vi "SP Convert 3.0 - 3.1 to 3.2 and 4.0 - 4.1.vi"(1 "S Parameter 3.0 - 3.1 Test Parameters":T2={"Tag"="", "Stimulus"={"Use Instrument Settings"=FALSE, "Sweep Type"=enum."Linear", "Sweep"=[{"Fstart, MHz"=500.0, "Fstop, MHz"=1500.0, "Points"=201}], "Blank Frequencies"=FALSE, "Power, dBm"=999.0, "IFBW, Hz"=-1.0, "Sweep Time, s"=-1.0}, "Measurements"=[{"Parameter"=enum."S11", "Channel"=1, "Limits"=[]}], "Reports"={"Reports to Generate"=[], "Print Reports"=FALSE}, "Quick Mode"=FALSE, "Display"={"Retain Settings"=FALSE, "Lock Control"=FALSE, "Plot Orientation"=enum."Single", "CH Controls"=[{"Trace Orientation"=enum."Overlay", "Frequency"={"Start"=500.0, "Stop"=1500.0, "Units"="MHz"}, "CH1Control"={"ChOn"=TRUE, "Measure"=0, "Format"=0, "Autoscale"=TRUE, "Reference"=0.0, "\nRefUnit"="dB/Div", "Position"=5.0, "Scale"=10.0, "ScaleUnit"="dB/Div", "LimitOn"=TRUE, "LimitFill"=FALSE, "Display Data"=0, "Show Markers"=FALSE}, "CH2Control"={"ChOn"=TRUE, "Measure"=0, "Format"=0, "Autoscale"=TRUE, "Reference"=0.0, "\nRefUnit"="dB/Div", "Position"=5.0, "Scale"=10.0, "ScaleUnit"="dB/Div", "LimitOn"=TRUE, "LimitFill"=FALSE, "Display Data"=0, "Show Markers"=FALSE}, "Markers"=[]}, {"Trace Orientation"=enum."Overlay", "Frequency"={"Start"=500.0, "Stop"=1500.0, "Units"="MHz"}, "CH1Control"={"ChOn"=TRUE, "Measure"=0, "Format"=0, "Autoscale"=TRUE, "Reference"=0.0, "\nRefUnit"="dB/Div", "Position"=5.0, "Scale"=10.0, "ScaleUnit"="dB/Div", "LimitOn"=TRUE, "LimitFill"=FALSE, "Display Data"=0, "Show Markers"=FALSE}, "CH2Control"={"ChOn"=TRUE, "Measure"=0, "Format"=0, "Autoscale"=TRUE, "Reference"=0.0, "\nRefUnit"="dB/Div", "Position"=5.0, "Scale"=10.0, "ScaleUnit"="dB/Div", "LimitOn"=TRUE, "LimitFill"=FALSE, "Display Data"=0, "Show Markers"=FALSE}, "Markers"=[]}, {"Trace Orientation"=enum."Overlay", "Frequency"={"Start"=500.0, "Stop"=1500.0, "Units"="MHz"}, "CH1Control"={"ChOn"=TRUE, "Measure"=0, "Format"=0, "Autoscale"=TRUE, "Reference"=0.0, "\nRefUnit"="dB/Div", "Position"=5.0, "Scale"=10.0, "ScaleUnit"="dB/Div", "LimitOn"=TRUE, "LimitFill"=FALSE, "Display Data"=0, "Show Markers"=FALSE}, "CH2Control"={"ChOn"=TRUE, "Measure"=0, "Format"=0, "Autoscale"=TRUE, "Reference"=0.0, "\nRefUnit"="dB/Div", "Position"=5.0, "Scale"=10.0, "ScaleUnit"="dB/Div", "LimitOn"=TRUE, "LimitFill"=FALSE, "Display Data"=0, "Show Markers"=FALSE}, "Markers"=[]}, {"Trace Orientation"=enum."Overlay", "Frequency"={"Start"=500.0, "Stop"=1500.0, "Units"="MHz"}, "CH1Control"={"ChOn"=TRUE, "Measure"=0, "Format"=0, "Autoscale"=TRUE, "Reference"=0.0, "\nRefUnit"="dB/Div", "Position"=5.0, "Scale"=10.0, "ScaleUnit"="dB/Div", "LimitOn"=TRUE, "LimitFill"=FALSE, "Display Data"=0, "Show Markers"=FALSE}, "CH2Control"={"ChOn"=TRUE, "Measure"=0, "Format"=0, "Autoscale"=TRUE, "Reference"=0.0, "\nRefUnit"="dB/Div", "Position"=5.0, "Scale"=10.0, "ScaleUnit"="dB/Div", "LimitOn"=TRUE, "LimitFill"=FALSE, "Display Data"=0, "Show Markers"=FALSE}, "Markers"=[]}], "Formatted Data"=FALSE}, "Calibrations"=[enum."Not Calibrated", enum."Not Calibrated", enum."Not Calibrated", enum."Not Calibrated"]} {"Stimulus"."Sweep Time, s" format="%.3g"; "Display"."CH Controls"."Frequency"."Stop" format="%.3g"; "Display"."CH Controls"."Frequency"."Start" format="%.3g"; "Display"."CH Controls"."CH2Control"."Measure" items=["S11", "S21", "S12", "S22"]; "Display"."CH Controls"."CH2Control"."Reference" format="%#.2g"; "Display"."CH Controls"."CH2Control"."Display Data" items=["Data", "Memory", "Data/Memory"]; "Display"."CH Controls"."CH2Control"."Format" items=["Log Mag", "Phase", "Delay", "Smith", "Polar", "Lin Mag", "SWR", "Loss", "Real", "Imaginary"]; "Display"."CH Controls"."CH2Control"."Scale" min=0.001 step=1.0 format="%#.2g"; "Display"."CH Controls"."CH2Control"."Position" min=0.0 max=10.0; "Display"."CH Controls"."CH1Control"."Measure" items=["S11", "S21", "S12", "S22"]; "Display"."CH Controls"."CH1Control"."Reference" format="%#.2g"; "Display"."CH Controls"."CH1Control"."Display Data" items=["Data", "Memory", "Data/Memory"]; "Display"."CH Controls"."CH1Control"."Format" items=["Log Mag", "Phase", "Delay", "Smith", "Polar", "Lin Mag", "SWR", "Loss", "Real", "Imaginary"]; "Display"."CH Controls"."CH1Control"."Scale" min=0.001 step=1.0 format="%#.2g"; "Display"."CH Controls"."CH1Control"."Position" min=0.0 max=10.0; "Measurements"."Channel" min=1 max=99 step=1; "Measurements"."Limits"."Run" min=1 step=1}) -> (0 "S Parameter 3.2 - 4.1 Test Parameters":T1={"Tag"="", "Stimulus"={"Use Instrument Settings"=FALSE, "Sweep Type"=enum."Linear", "Sweep"=[{"Fstart, MHz"=500.0, "Fstop, MHz"=1500.0, "Points"=201}], "Blank Frequencies"=FALSE, "Power, dBm"=999.0, "IFBW, Hz"=-1.0, "Sweep Time, s"=-1.0}, "Measurements"=[], "Datasheets"={"Datasheets to Generate"=[], "Print Datasheets"=FALSE}, "Quick Mode"=FALSE, "Display"={"Retain Settings"=TRUE, "Lock Control"=FALSE, "Plot Orientation"=enum."Single", "CH Controls"=[{"Trace Orientation"=enum."Overlay", "Frequency"={"Start"=500.0, "Stop"=1500.0, "Units"="MHz"}, "CH1Control"={"ChOn"=TRUE, "Measure"=0, "Format"=6, "Autoscale"=FALSE, "Reference"=0.0, "\nRefUnit"="dB/Div", "Position"=5.0, "Scale"=1.0, "ScaleUnit"="dB/Div", "LimitOn"=TRUE, "LimitFill"=FALSE, "Display Data"=0, "Show Markers"=FALSE, "SXX"=""}, "CH2Control"={"ChOn"=TRUE, "Measure"=0, "Format"=6, "Autoscale"=FALSE, "Reference"=0.0, "\nRefUnit"="dB/Div", "Position"=5.0, "Scale"=1.0, "ScaleUnit"="dB/Div", "LimitOn"=TRUE, "LimitFill"=FALSE, "Display Data"=0, "Show Markers"=FALSE, "SXX"=""}, "Markers"=[]}, {"Trace Orientation"=enum."Overlay", "Frequency"={"Start"=500.0, "Stop"=1500.0, "Units"="MHz"}, "CH1Control"={"ChOn"=TRUE, "Measure"=0, "Format"=6, "Autoscale"=TRUE, "Reference"=0.0, "\nRefUnit"="dB/Div", "Position"=5.0, "Scale"=1.0, "ScaleUnit"="dB/Div", "LimitOn"=TRUE, "LimitFill"=FALSE, "Display Data"=0, "Show Markers"=FALSE, "SXX"=""}, "CH2Control"={"ChOn"=TRUE, "Measure"=1, "Format"=0, "Autoscale"=TRUE, "Reference"=0.0, "\nRefUnit"="dB/Div", "Position"=5.0, "Scale"=1.0, "ScaleUnit"="dB/Div", "LimitOn"=TRUE, "LimitFill"=FALSE, "Display Data"=0, "Show Markers"=FALSE, "SXX"=""}, "Markers"=[]}, {"Trace Orientation"=enum."Overlay", "Frequency"={"Start"=500.0, "Stop"=1500.0, "Units"="MHz"}, "CH1Control"={"ChOn"=TRUE, "Measure"=0, "Format"=6, "Autoscale"=TRUE, "Reference"=0.0, "\nRefUnit"="dB/Div", "Position"=5.0, "Scale"=1.0, "ScaleUnit"="dB/Div", "LimitOn"=TRUE, "LimitFill"=FALSE, "Display Data"=0, "Show Markers"=FALSE, "SXX"=""}, "CH2Control"={"ChOn"=TRUE, "Measure"=1, "Format"=0, "Autoscale"=TRUE, "Reference"=0.0, "\nRefUnit"="dB/Div", "Position"=5.0, "Scale"=1.0, "ScaleUnit"="dB/Div", "LimitOn"=TRUE, "LimitFill"=FALSE, "Display Data"=0, "Show Markers"=FALSE, "SXX"=""}, "Markers"=[]}, {"Trace Orientation"=enum."Overlay", "Frequency"={"Start"=500.0, "Stop"=1500.0, "Units"="MHz"}, "CH1Control"={"ChOn"=TRUE, "Measure"=0, "Format"=6, "Autoscale"=TRUE, "Reference"=0.0, "\nRefUnit"="dB/Div", "Position"=5.0, "Scale"=1.0, "ScaleUnit"="dB/Div", "LimitOn"=TRUE, "LimitFill"=FALSE, "Display Data"=0, "Show Markers"=FALSE, "SXX"=""}, "CH2Control"={"ChOn"=TRUE, "Measure"=1, "Format"=0, "Autoscale"=TRUE, "Reference"=0.0, "\nRefUnit"="dB/Div", "Position"=5.0, "Scale"=1.0, "ScaleUnit"="dB/Div", "LimitOn"=TRUE, "LimitFill"=FALSE, "Display Data"=0, "Show Markers"=FALSE, "SXX"=""}, "Markers"=[]}], "Formatted Data"=FALSE}, "Auto Select"=TRUE, "Calibration"={"State"=FALSE, "String"=""}} {"Stimulus"."Sweep Time, s" format="%.3g"; "Display"."CH Controls"."Frequency"."Stop" format="%.3g"; "Display"."CH Controls"."Frequency"."Start" format="%.3g"; "Display"."CH Controls"."CH2Control"."Reference" format="%#.2g"; "Display"."CH Controls"."CH2Control"."Display Data" items=["Data", "Memory", "Data/Memory"]; "Display"."CH Controls"."CH2Control"."Format" items=["Log Mag", "Phase", "Delay", "Smith", "Polar", "Lin Mag", "SWR", "Loss", "Real", "Imaginary"]; "Display"."CH Controls"."CH2Control"."Scale" min=0.001 step=1.0 format="%#.2g"; "Display"."CH Controls"."CH2Control"."Position" min=0.0 max=10.0; "Display"."CH Controls"."CH1Control"."Reference" format="%#.2g"; "Display"."CH Controls"."CH1Control"."Display Data" items=["Data", "Memory", "Data/Memory"]; "Display"."CH Controls"."CH1Control"."Format" items=["Log Mag", "Phase", "Delay", "Smith", "Polar", "Lin Mag", "SWR", "Loss", "Real", "Imaginary"]; "Display"."CH Controls"."CH1Control"."Scale" min=0.001 step=1.0 format="%#.2g"; "Display"."CH Controls"."CH1Control"."Position" min=0.0 max=10.0; "Measurements"."Parameters"."Limits"."Run" min=1 step=1; "Measurements"."Channel" min=0 max=32 step=1})   [LabVIEW 2011]
uses:
  TypeDefs/SP Test Parameters v3.0-3.1.ctl
  TypeDefs/SP Test Parameters v3.2 and 4.0-4.1.ctl
  TypeDefs/SP Parameter.ctl
panel:
  # "Div"
  # "Div"
  # "="
  # "Div"
  # "Div"
  # "="
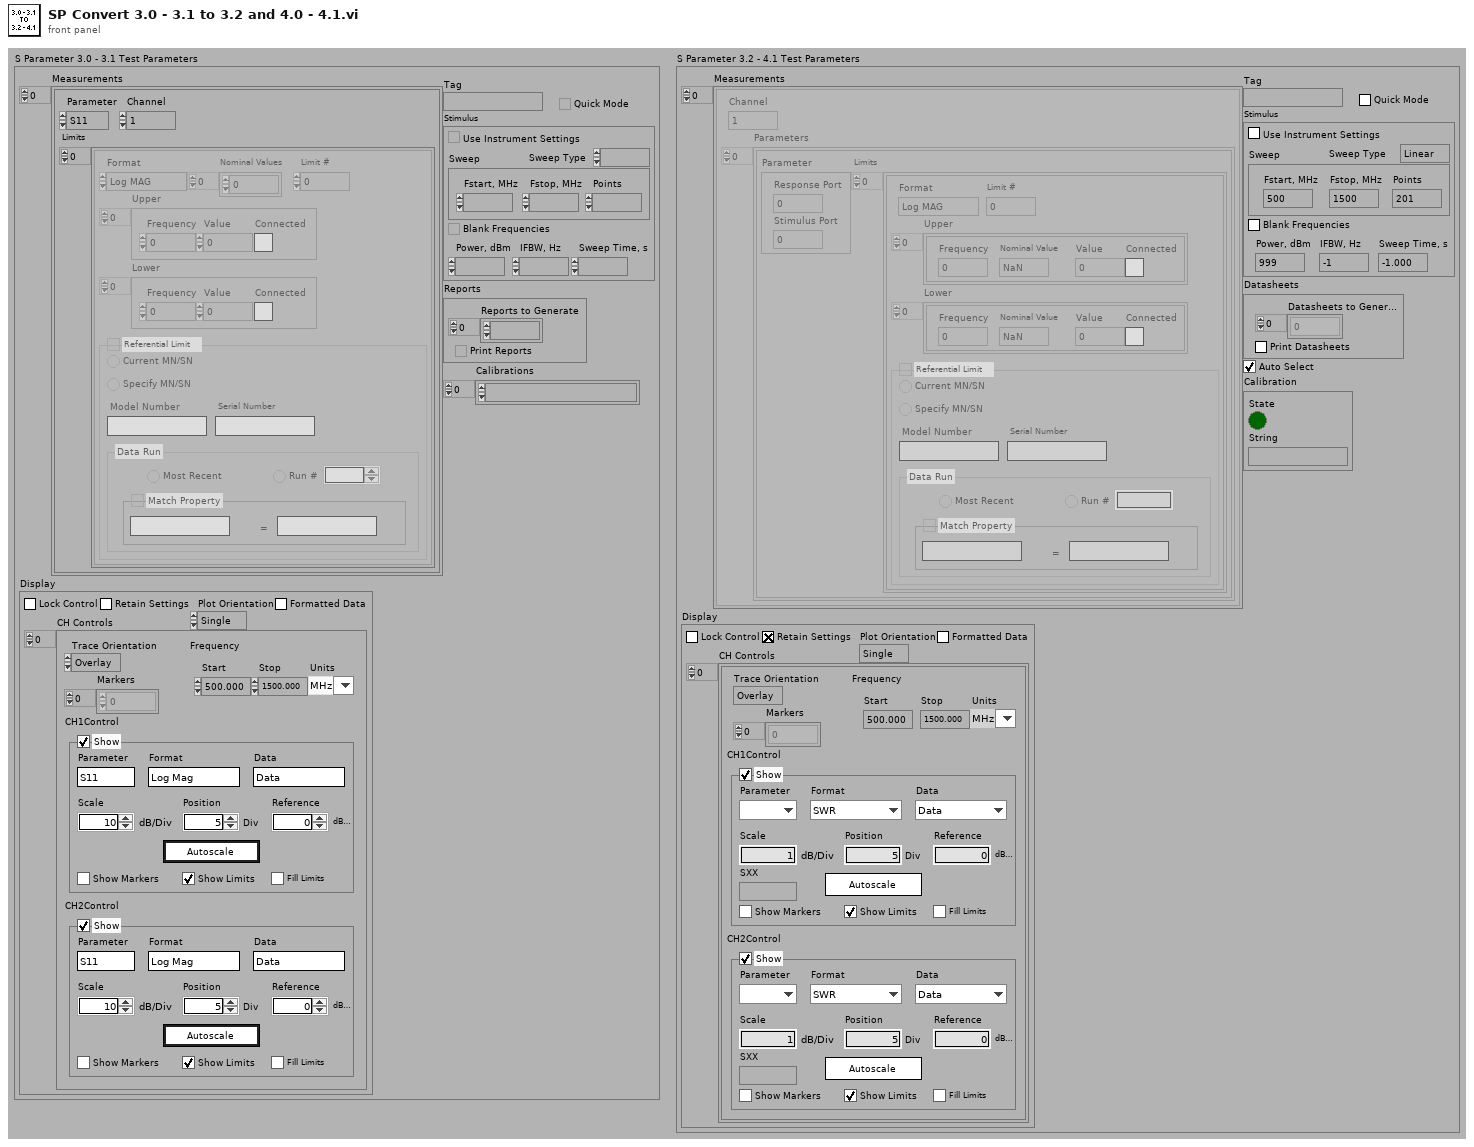
[diagram p1: front panel]
types:
  T1 = typedef "SP Test Parameters v3.2 and 4.0-4.1.ctl" = cluster{"Tag":string, "Stimulus":cluster{"Use Instrument Settings":bool, "Sweep Type":enum32{"Linear", "Log", "List", "Power", "CW"}, "Sweep":cluster{"Fstart, MHz":dbl, "Fstop, MHz":dbl, "Points":i32}[], "Blank Frequencies":bool, "Power, dBm":dbl, "IFBW, Hz":dbl, "Sweep Time, s":dbl}, "Measurements":cluster{"Channel":i8, "Parameters":cluster{"Parameter":cluster{"Stimulus Port":i8, "Response Port":i8}, "Limits":cluster{"Format":enum16{"Log MAG", "Lin MAG", "VSWR", "Phase", "Delay", "Insertion Loss", "Isolation", "Return Loss"}, "Upper":cluster{"Frequency":dbl, "Nominal Value":dbl, "Value":dbl, "Connected":bool}[], "Lower":cluster{"Frequency":dbl, "Nominal Value":dbl, "Value":dbl, "Connected":bool}[], "Limit #":i32, "Ref Limit":bool, "Ref Type":enum32{"Current", "Specify"}, "Model":string, "Serial":string, "Run Type":enum32{"Most Recent", "Run #"}, "Run":i32, "Match Property":bool, "Property":string, "Property Value":string}[]}[]}[], "Datasheets":cluster{"Datasheets to Generate":i32[], "Print Datasheets":bool}, "Quick Mode":bool, "Display":cluster{"Retain Settings":bool, "Lock Control":bool, "Plot Orientation":enum32{"Single", "Dual", "Quad"}, "CH Controls":cluster{"Trace Orientation":enum32{"Overlay", "Split"}, "Frequency":cluster{"Start":dbl, "Stop":dbl, "Units":string}, "CH1Control":cluster{"ChOn":bool, "Measure":i32, "Format":i32, "Autoscale":bool, "Reference":dbl, "\nRefUnit":string, "Position":dbl, "Scale":dbl, "ScaleUnit":string, "LimitOn":bool, "LimitFill":bool, "Display Data":u16, "Show Markers":bool, "SXX":string}, "CH2Control":cluster{"ChOn":bool, "Measure":i32, "Format":i32, "Autoscale":bool, "Reference":dbl, "\nRefUnit":string, "Position":dbl, "Scale":dbl, "ScaleUnit":string, "LimitOn":bool, "LimitFill":bool, "Display Data":u16, "Show Markers":bool, "SXX":string}, "Markers":dbl[]}[], "Formatted Data":bool}, "Auto Select":bool, "Calibration":cluster{"State":bool, "String":string}}
  T2 = typedef "SP Test Parameters v3.0-3.1.ctl" = cluster{"Tag":string, "Stimulus":cluster{"Use Instrument Settings":bool, "Sweep Type":enum32{"Linear", "Log", "List", "Power", "CW"}, "Sweep":cluster{"Fstart, MHz":dbl, "Fstop, MHz":dbl, "Points":i32}[], "Blank Frequencies":bool, "Power, dBm":dbl, "IFBW, Hz":dbl, "Sweep Time, s":dbl}, "Measurements":cluster{"Parameter":enum32{"S11", "S21", "S12", "S22"}, "Channel":i32, "Limits":cluster{"Format":enum16{"Log MAG", "Lin MAG", "VSWR", "Phase", "Delay", "Insertion Loss", "Isolation", "Return Loss"}, "Upper":cluster{"Frequency":dbl, "Value":dbl, "Connected":bool}[], "Lower":cluster{"Frequency":dbl, "Value":dbl, "Connected":bool}[], "Nominal Values":dbl[], "Limit #":i32, "Ref Limit":bool, "Ref Type":enum32{"Current", "Specify"}, "Model":string, "Serial":string, "Run Type":enum32{"Most Recent", "Run #"}, "Run":i32, "Match Property":bool, "Property":string, "Property Value":string}[]}[], "Reports":cluster{"Reports to Generate":i32[], "Print Reports":bool}, "Quick Mode":bool, "Display":cluster{"Retain Settings":bool, "Lock Control":bool, "Plot Orientation":enum32{"Single", "Dual", "Quad"}, "CH Controls":cluster{"Trace Orientation":enum32{"Overlay", "Split"}, "Frequency":cluster{"Start":dbl, "Stop":dbl, "Units":string}, "CH1Control":cluster{"ChOn":bool, "Measure":i32, "Format":i32, "Autoscale":bool, "Reference":dbl, "\nRefUnit":string, "Position":dbl, "Scale":dbl, "ScaleUnit":string, "LimitOn":bool, "LimitFill":bool, "Display Data":u16, "Show Markers":bool}, "CH2Control":cluster{"ChOn":bool, "Measure":i32, "Format":i32, "Autoscale":bool, "Reference":dbl, "\nRefUnit":string, "Position":dbl, "Scale":dbl, "ScaleUnit":string, "LimitOn":bool, "LimitFill":bool, "Display Data":u16, "Show Markers":bool}, "Markers":dbl[]}[], "Formatted Data":bool}, "Calibrations":enum32{"Not Calibrated", "Response", "Response and Isolation", "Full 1-Port (Port 1)", "Full 1-Port (Port 2)", "Full 2-Port", "One Path 2-Port", "TRL/LRM  2-Port", "TOSM Multi-Port", "TOM 2-Port", "TRM 2-Port", "TNA 2-Port"}[]}
  T3 = enum32{"Not Calibrated", "Response", "Response and Isolation", "Full 1-Port (Port 1)", "Full 1-Port (Port 2)", "Full 2-Port", "One Path 2-Port", "TRL/LRM  2-Port", "TOSM Multi-Port", "TOM 2-Port", "TRM 2-Port", "TNA 2-Port"}
  T4 = cluster{"Trace Orientation":enum32{"Overlay", "Split"}, "Frequency":cluster{"Start":dbl, "Stop":dbl, "Units":string}, "CH1Control":cluster{"ChOn":bool, "Measure":i32, "Format":i32, "Autoscale":bool, "Reference":dbl, "\nRefUnit":string, "Position":dbl, "Scale":dbl, "ScaleUnit":string, "LimitOn":bool, "LimitFill":bool, "Display Data":u16, "Show Markers":bool, "SXX":string}, "CH2Control":cluster{"ChOn":bool, "Measure":i32, "Format":i32, "Autoscale":bool, "Reference":dbl, "\nRefUnit":string, "Position":dbl, "Scale":dbl, "ScaleUnit":string, "LimitOn":bool, "LimitFill":bool, "Display Data":u16, "Show Markers":bool, "SXX":string}, "Markers":dbl[]}[]
  T5 = cluster{"Channel":i8, "Parameters":cluster{"Parameter":cluster{"Stimulus Port":i8, "Response Port":i8}, "Limits":cluster{"Format":enum16{"Log MAG", "Lin MAG", "VSWR", "Phase", "Delay", "Insertion Loss", "Isolation", "Return Loss"}, "Upper":cluster{"Frequency":dbl, "Nominal Value":dbl, "Value":dbl, "Connected":bool}[], "Lower":cluster{"Frequency":dbl, "Nominal Value":dbl, "Value":dbl, "Connected":bool}[], "Limit #":i32, "Ref Limit":bool, "Ref Type":enum32{"Current", "Specify"}, "Model":string, "Serial":string, "Run Type":enum32{"Most Recent", "Run #"}, "Run":i32, "Match Property":bool, "Property":string, "Property Value":string}[]}[]}[]
  T6 = cluster{"Use Instrument Settings":bool, "Sweep Type":enum32{"Linear", "Log", "List", "Power", "CW"}, "Sweep":cluster{"Fstart, MHz":dbl, "Fstop, MHz":dbl, "Points":i32}[], "Blank Frequencies":bool, "Power, dBm":dbl, "IFBW, Hz":dbl, "Sweep Time, s":dbl}
  T7 = cluster{"Reports to Generate":i32[], "Print Reports":bool}
  T8 = enum32{"Not Calibrated", "Response", "Response and Isolation", "Full 1-Port (Port 1)", "Full 1-Port (Port 2)", "Full 2-Port", "One Path 2-Port", "TRL/LRM  2-Port", "TOSM Multi-Port", "TOM 2-Port", "TRM 2-Port", "TNA 2-Port"}[]
  T9 = cluster{"Trace Orientation":enum32{"Overlay", "Split"}, "Frequency":cluster{"Start":dbl, "Stop":dbl, "Units":string}, "CH1Control":cluster{"ChOn":bool, "Measure":i32, "Format":i32, "Autoscale":bool, "Reference":dbl, "\nRefUnit":string, "Position":dbl, "Scale":dbl, "ScaleUnit":string, "LimitOn":bool, "LimitFill":bool, "Display Data":u16, "Show Markers":bool}, "CH2Control":cluster{"ChOn":bool, "Measure":i32, "Format":i32, "Autoscale":bool, "Reference":dbl, "\nRefUnit":string, "Position":dbl, "Scale":dbl, "ScaleUnit":string, "LimitOn":bool, "LimitFill":bool, "Display Data":u16, "Show Markers":bool}, "Markers":dbl[]}[]
  T10 = cluster{"Parameter":enum32{"S11", "S21", "S12", "S22"}, "Channel":i32, "Limits":cluster{"Format":enum16{"Log MAG", "Lin MAG", "VSWR", "Phase", "Delay", "Insertion Loss", "Isolation", "Return Loss"}, "Upper":cluster{"Frequency":dbl, "Value":dbl, "Connected":bool}[], "Lower":cluster{"Frequency":dbl, "Value":dbl, "Connected":bool}[], "Nominal Values":dbl[], "Limit #":i32, "Ref Limit":bool, "Ref Type":enum32{"Current", "Specify"}, "Model":string, "Serial":string, "Run Type":enum32{"Most Recent", "Run #"}, "Run":i32, "Match Property":bool, "Property":string, "Property Value":string}[]}[]
  T11 = cluster{"Channel":i8, "Parameters":cluster{"Parameter":cluster{"Stimulus Port":i8, "Response Port":i8}, "Limits":cluster{"Format":enum16{"Log MAG", "Lin MAG", "VSWR", "Phase", "Delay", "Insertion Loss", "Isolation", "Return Loss"}, "Upper":cluster{"Frequency":dbl, "Nominal Value":dbl, "Value":dbl, "Connected":bool}[], "Lower":cluster{"Frequency":dbl, "Nominal Value":dbl, "Value":dbl, "Connected":bool}[], "Limit #":i32, "Ref Limit":bool, "Ref Type":enum32{"Current", "Specify"}, "Model":string, "Serial":string, "Run Type":enum32{"Most Recent", "Run #"}, "Run":i32, "Match Property":bool, "Property":string, "Property Value":string}[]}[]}
  T12 = cluster{"Parameter":cluster{"Stimulus Port":i8, "Response Port":i8}, "Limits":cluster{"Format":enum16{"Log MAG", "Lin MAG", "VSWR", "Phase", "Delay", "Insertion Loss", "Isolation", "Return Loss"}, "Upper":cluster{"Frequency":dbl, "Nominal Value":dbl, "Value":dbl, "Connected":bool}[], "Lower":cluster{"Frequency":dbl, "Nominal Value":dbl, "Value":dbl, "Connected":bool}[], "Limit #":i32, "Ref Limit":bool, "Ref Type":enum32{"Current", "Specify"}, "Model":string, "Serial":string, "Run Type":enum32{"Most Recent", "Run #"}, "Run":i32, "Match Property":bool, "Property":string, "Property Value":string}[]}[]
  T13 = cluster{"Trace Orientation":enum32{"Overlay", "Split"}, "Frequency":cluster{"Start":dbl, "Stop":dbl, "Units":string}, "CH1Control":cluster{"ChOn":bool, "Measure":i32, "Format":i32, "Autoscale":bool, "Reference":dbl, "\nRefUnit":string, "Position":dbl, "Scale":dbl, "ScaleUnit":string, "LimitOn":bool, "LimitFill":bool, "Display Data":u16, "Show Markers":bool, "SXX":string}, "CH2Control":cluster{"ChOn":bool, "Measure":i32, "Format":i32, "Autoscale":bool, "Reference":dbl, "\nRefUnit":string, "Position":dbl, "Scale":dbl, "ScaleUnit":string, "LimitOn":bool, "LimitFill":bool, "Display Data":u16, "Show Markers":bool, "SXX":string}, "Markers":dbl[]}
  T14 = typedef "SP Display Data.ctl" = u16
  T15 = cluster{"Parameter":cluster{"Stimulus Port":i8, "Response Port":i8}, "Limits":cluster{"Format":enum16{"Log MAG", "Lin MAG", "VSWR", "Phase", "Delay", "Insertion Loss", "Isolation", "Return Loss"}, "Upper":cluster{"Frequency":dbl, "Nominal Value":dbl, "Value":dbl, "Connected":bool}[], "Lower":cluster{"Frequency":dbl, "Nominal Value":dbl, "Value":dbl, "Connected":bool}[], "Limit #":i32, "Ref Limit":bool, "Ref Type":enum32{"Current", "Specify"}, "Model":string, "Serial":string, "Run Type":enum32{"Most Recent", "Run #"}, "Run":i32, "Match Property":bool, "Property":string, "Property Value":string}[]}
  T16 = cluster{"Format":enum16{"Log MAG", "Lin MAG", "VSWR", "Phase", "Delay", "Insertion Loss", "Isolation", "Return Loss"}, "Upper":cluster{"Frequency":dbl, "Nominal Value":dbl, "Value":dbl, "Connected":bool}[], "Lower":cluster{"Frequency":dbl, "Nominal Value":dbl, "Value":dbl, "Connected":bool}[], "Limit #":i32, "Ref Limit":bool, "Ref Type":enum32{"Current", "Specify"}, "Model":string, "Serial":string, "Run Type":enum32{"Most Recent", "Run #"}, "Run":i32, "Match Property":bool, "Property":string, "Property Value":string}[]
  T17 = cluster{"Format":enum16{"Log MAG", "Lin MAG", "VSWR", "Phase", "Delay", "Insertion Loss", "Isolation", "Return Loss"}, "Upper":cluster{"Frequency":dbl, "Nominal Value":dbl, "Value":dbl, "Connected":bool}[], "Lower":cluster{"Frequency":dbl, "Nominal Value":dbl, "Value":dbl, "Connected":bool}[], "Limit #":i32, "Ref Limit":bool, "Ref Type":enum32{"Current", "Specify"}, "Model":string, "Serial":string, "Run Type":enum32{"Most Recent", "Run #"}, "Run":i32, "Match Property":bool, "Property":string, "Property Value":string}
  T18 = cluster{"Frequency":dbl, "Nominal Value":dbl, "Value":dbl, "Connected":bool}[]
  T19 = cluster{"Frequency":dbl, "Nominal Value":dbl, "Value":dbl, "Connected":bool}
  T20 = typedef "SP Parameter.ctl" = cluster{"Stimulus Port":i8, "Response Port":i8}
  T21 = cluster{"Format":enum16{"Log MAG", "Lin MAG", "VSWR", "Phase", "Delay", "Insertion Loss", "Isolation", "Return Loss"}, "Upper":cluster{"Frequency":dbl, "Value":dbl, "Connected":bool}[], "Lower":cluster{"Frequency":dbl, "Value":dbl, "Connected":bool}[], "Nominal Values":dbl[], "Limit #":i32, "Ref Limit":bool, "Ref Type":enum32{"Current", "Specify"}, "Model":string, "Serial":string, "Run Type":enum32{"Most Recent", "Run #"}, "Run":i32, "Match Property":bool, "Property":string, "Property Value":string}[]
  T22 = enum16{"Log MAG", "Lin MAG", "VSWR", "Phase", "Delay", "Insertion Loss", "Isolation", "Return Loss"}
  T23 = cluster{"Frequency":dbl, "Value":dbl, "Connected":bool}[]
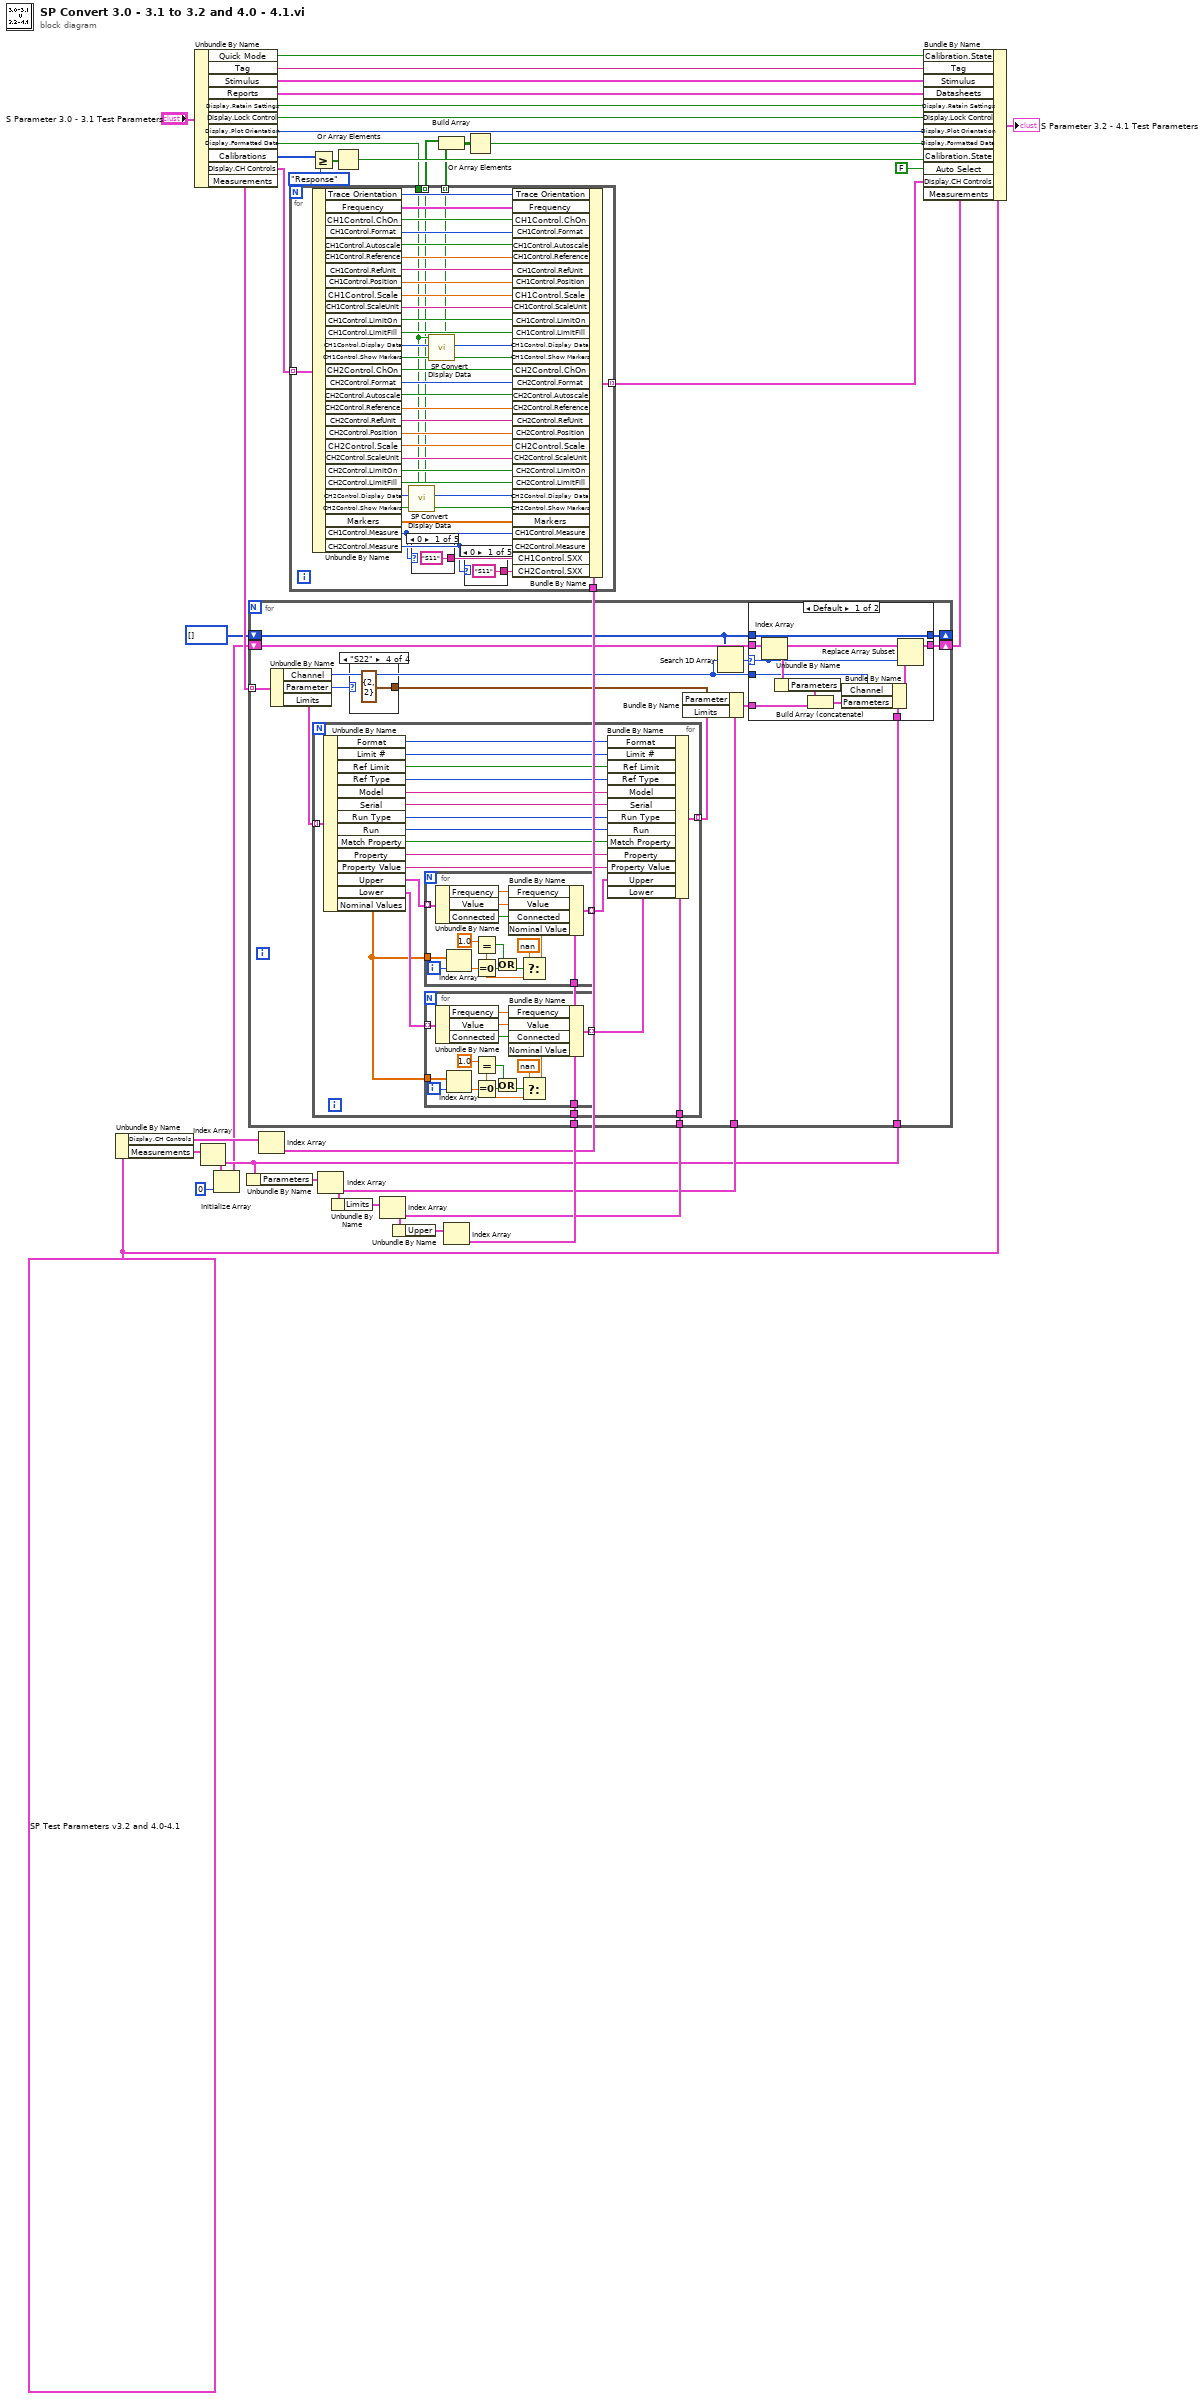
[diagram p0: block diagram]
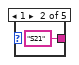
[diagram p2: hidden frame]
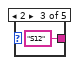
[diagram p3: hidden frame]
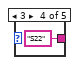
[diagram p4: hidden frame]
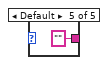
[diagram p5: hidden frame]
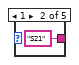
[diagram p6: hidden frame]
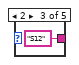
[diagram p7: hidden frame]
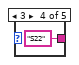
[diagram p8: hidden frame]
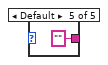
[diagram p9: hidden frame]
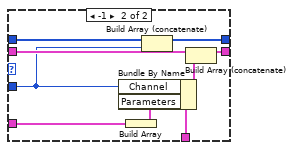
[diagram p10: hidden frame]
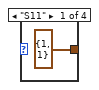
[diagram p11: hidden frame]
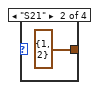
[diagram p12: hidden frame]
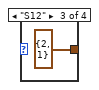
[diagram p13: hidden frame]
diagram:
  w8 = T1 {"Tag"="", "Stimulus"={"Use Instrument Settings"=FALSE, "Sweep Type"=enum."Linear", "Sweep"=[{"Fstart, MHz"=500.0, "Fstop, MHz"=1500.0, "Points"=201}], "Blank Frequencies"=FALSE, "Power, dBm"=999.0, "IFBW, Hz"=-1.0, "Sweep Time, s"=-1.0}, "Measurements"=[], "Datasheets"={"Datasheets to Generate"=[], "Print Datasheets"=FALSE}, "Quick Mode"=FALSE, "Display"={"Retain Settings"=TRUE, "Lock Control"=FALSE, "Plot Orientation"=enum."Single", "CH Controls"=[{"Trace Orientation"=enum."Overlay", "Frequency"={"Start"=500.0, "Stop"=1500.0, "Units"="MHz"}, "CH1Control"={"ChOn"=TRUE, "Measure"=0, "Format"=6, "Autoscale"=FALSE, "Reference"=0.0, "\nRefUnit"="dB/Div", "Position"=5.0, "Scale"=1.0, "ScaleUnit"="dB/Div", "LimitOn"=TRUE, "LimitFill"=FALSE, "Display Data"=0, "Show Markers"=FALSE, "SXX"=""}, "CH2Control"={"ChOn"=TRUE, "Measure"=0, "Format"=6, "Autoscale"=FALSE, "Reference"=0.0, "\nRefUnit"="dB/Div", "Position"=5.0, "Scale"=1.0, "ScaleUnit"="dB/Div", "LimitOn"=TRUE, "LimitFill"=FALSE, "Display Data"=0, "Show Markers"=FALSE, "SXX"=""}, "Markers"=[]}, {"Trace Orientation"=enum."Overlay", "Frequency"={"Start"=500.0, "Stop"=1500.0, "Units"="MHz"}, "CH1Control"={"ChOn"=TRUE, "Measure"=0, "Format"=6, "Autoscale"=TRUE, "Reference"=0.0, "\nRefUnit"="dB/Div", "Position"=5.0, "Scale"=1.0, "ScaleUnit"="dB/Div", "LimitOn"=TRUE, "LimitFill"=FALSE, "Display Data"=0, "Show Markers"=FALSE, "SXX"=""}, "CH2Control"={"ChOn"=TRUE, "Measure"=1, "Format"=0, "Autoscale"=TRUE, "Reference"=0.0, "\nRefUnit"="dB/Div", "Position"=5.0, "Scale"=1.0, "ScaleUnit"="dB/Div", "LimitOn"=TRUE, "LimitFill"=FALSE, "Display Data"=0, "Show Markers"=FALSE, "SXX"=""}, "Markers"=[]}, {"Trace Orientation"=enum."Overlay", "Frequency"={"Start"=500.0, "Stop"=1500.0, "Units"="MHz"}, "CH1Control"={"ChOn"=TRUE, "Measure"=0, "Format"=6, "Autoscale"=TRUE, "Reference"=0.0, "\nRefUnit"="dB/Div", "Position"=5.0, "Scale"=1.0, "ScaleUnit"="dB/Div", "LimitOn"=TRUE, "LimitFill"=FALSE, "Display Data"=0, "Show Markers"=FALSE, "SXX"=""}, "CH2Control"={"ChOn"=TRUE, "Measure"=1, "Format"=0, "Autoscale"=TRUE, "Reference"=0.0, "\nRefUnit"="dB/Div", "Position"=5.0, "Scale"=1.0, "ScaleUnit"="dB/Div", "LimitOn"=TRUE, "LimitFill"=FALSE, "Display Data"=0, "Show Markers"=FALSE, "SXX"=""}, "Markers"=[]}, {"Trace Orientation"=enum."Overlay", "Frequency"={"Start"=500.0, "Stop"=1500.0, "Units"="MHz"}, "CH1Control"={"ChOn"=TRUE, "Measure"=0, "Format"=6, "Autoscale"=TRUE, "Reference"=0.0, "\nRefUnit"="dB/Div", "Position"=5.0, "Scale"=1.0, "ScaleUnit"="dB/Div", "LimitOn"=TRUE, "LimitFill"=FALSE, "Display Data"=0, "Show Markers"=FALSE, "SXX"=""}, "CH2Control"={"ChOn"=TRUE, "Measure"=1, "Format"=0, "Autoscale"=TRUE, "Reference"=0.0, "\nRefUnit"="dB/Div", "Position"=5.0, "Scale"=1.0, "ScaleUnit"="dB/Div", "LimitOn"=TRUE, "LimitFill"=FALSE, "Display Data"=0, "Show Markers"=FALSE, "SXX"=""}, "Markers"=[]}], "Formatted Data"=FALSE}, "Auto Select"=TRUE, "Calibration"={"State"=FALSE, "String"=""}} ("S Parameter Test Parameters")
  n1 = Unbundle By Name(w8) -> ("Display.CH Controls"=w34:T4, "Measurements"=w32:T5)
  n2 = Unbundle By Name("S Parameter 3.0 - 3.1 Test Parameters") -> ("Quick Mode"=w27:bool, "Tag"=w31:string, "Stimulus"=w28:T6, "Reports"=w29:T7, "Display.Retain Settings"=w25:bool, "Display.Lock Control"=w24:bool, "Display.Plot Orientation"=w23:enum32{"Single", "Dual", "Quad"}, "Display.Formatted Data"=w5:bool, "Calibrations"=w26:T8, "Display.CH Controls"=w22:T9, "Measurements"=w30:T10)
  n3 = Index Array(array=w32) -> (element=w11:T11)  [unwired: 1 in]
  n4 = Initialize Array(w11, 0 ("dimension size")) -> (w9:T5)
  n5 = Unbundle By Name(w11) -> ("Parameters"=w35:T12)
  n6 = Index Array(array=w34) -> (element=w10:T13)  [unwired: 1 in]
  n7 = for {
    tunnel: w22 -> [w76] mode=indexing
    tunnel: w10 -> [w75]
    tunnel: [w72] -> w21 mode=indexing
    tunnel: w5 -> [w40]
    tunnel: [w39] -> w3 mode=indexing
    tunnel: [w38] -> w4 mode=indexing
    n8 = Unbundle By Name(w76) -> ("Trace Orientation"=w73:enum32{"Overlay", "Split"}, "Frequency"=w74:cluster{"Start":dbl, "Stop":dbl, "Units":string}, "CH1Control.ChOn"=w71:bool, "CH1Control.Format"=w70:i32, "CH1Control.Autoscale"=w69:bool, "CH1Control.Reference"=w68:dbl, "CH1Control.RefUnit"=w67:string, "CH1Control.Position"=w66:dbl, "CH1Control.Scale"=w65:dbl, "CH1Control.ScaleUnit"=w64:string, "CH1Control.LimitOn"=w63:bool, "CH1Control.LimitFill"=w62:bool, "CH1Control.Display Data"=w44:u16, "CH1Control.Show Markers"=w50:bool, "CH2Control.ChOn"=w61:bool, "CH2Control.Format"=w59:i32, "CH2Control.Autoscale"=w60:bool, "CH2Control.Reference"=w58:dbl, "CH2Control.RefUnit"=w57:string, "CH2Control.Position"=w56:dbl, "CH2Control.Scale"=w55:dbl, "CH2Control.ScaleUnit"=w54:string, "CH2Control.LimitOn"=w53:bool, "CH2Control.LimitFill"=w52:bool, "CH2Control.Display Data"=w42:u16, "CH2Control.Show Markers"=w51:bool, "Markers"=w49:dbl[], "CH1Control.Measure"=w45:i32, "CH2Control.Measure"=w46:i32)
    n9 = call "SP Convert Display Data.vi"("Old Formatted Data"=w40, "Old Data Display"=w42) -> ("New Data Display"=w41:T14, "New Formatted Data"=w38:bool)  [unwired: 8 out]
    n10 = case shown="0" w45 {
      tunnel: ["S11" ("CH1Control.SXX") "S21" ("CH1Control.SXX") "S12" ("CH1Control.SXX") "S22" ("CH1Control.SXX") "" ("CH1Control.SXX")] -> w48
      frame 0 {
      }
      frame 1 {
      }
      frame 2 {
      }
      frame 3 {
      }
      frame Default {
      }
    }
    n11 = call "SP Convert Display Data.vi"("Old Formatted Data"=w40, "Old Data Display"=w44) -> ("New Data Display"=w43:T14, "New Formatted Data"=w39:bool)  [unwired: 8 out]
    n12 = case shown="0" w46 {
      tunnel: ["S11" ("CH1Control.SXX") "S21" ("CH1Control.SXX") "S12" ("CH1Control.SXX") "S22" ("CH1Control.SXX") "" ("CH1Control.SXX")] -> w47
      frame 0 {
      }
      frame 1 {
      }
      frame 2 {
      }
      frame 3 {
      }
      frame Default {
      }
    }
    n13 = Bundle By Name(cluster=w75, "Trace Orientation"=w73, "Frequency"=w74, "CH1Control.ChOn"=w71, "CH1Control.Format"=w70, "CH1Control.Autoscale"=w69, "CH1Control.Reference"=w68, "CH1Control.RefUnit"=w67, "CH1Control.Position"=w66, "CH1Control.Scale"=w65, "CH1Control.ScaleUnit"=w64, "CH1Control.LimitOn"=w63, "CH1Control.LimitFill"=w62, "CH1Control.Display Data"=w43, "CH1Control.Show Markers"=w50, "CH2Control.ChOn"=w61, "CH2Control.Format"=w59, "CH2Control.Autoscale"=w60, "CH2Control.Reference"=w58, "CH2Control.RefUnit"=w57, "CH2Control.Position"=w56, "CH2Control.Scale"=w55, "CH2Control.ScaleUnit"=w54, "CH2Control.LimitOn"=w53, "CH2Control.LimitFill"=w52, "CH2Control.Display Data"=w41, "CH2Control.Show Markers"=w51, "Markers"=w49, "CH1Control.Measure"=w45, "CH2Control.Measure"=w46, "CH1Control.SXX"=w48, "CH2Control.SXX"=w47) -> (w72:T13)
  }
  n14 = Greater Or Equal?(x=w26, y=T3."Response" ("Calibration")) -> (x >= y?=w19:bool[])
  n15 = Index Array(array=w35) -> (element=w12:T15)  [unwired: 1 in]
  n16 = Unbundle By Name(w12) -> ("Limits"=w36:T16)
  n17 = Or Array Elements(Boolean array=w19) -> (logical OR=w18:bool)
  n18 = Index Array(array=w36) -> (element=w13:T17)  [unwired: 1 in]
  n19 = Unbundle By Name(w13) -> ("Upper"=w37:T18)
  n20 = Build Array(w4, w3) -> (w2:bool[][])
  n21 = Index Array(array=w37) -> (element=w14:T19)  [unwired: 1 in]
  n22 = for {
    tunnel: w30 -> [w102] mode=indexing
    tunnel: w11 -> [w101]
    tunnel: w13 -> [w99]
    tunnel: w14 -> [w98]
    tunnel: w12 -> [w97]
    shift-right: [w91] -> w7
    shift-left: w9 -> [w92]
    shift-right: [w90] -> _
    shift-left: i32[] [] -> [w89]
    n23 = Unbundle By Name(w102) -> ("Channel"=w88:i32, "Parameter"=w95:enum32{"S11", "S21", "S12", "S22"}, "Limits"=w100:T21)
    n24 = for {
      tunnel: w100 -> [w142] mode=indexing
      tunnel: w99 -> [w141]
      tunnel: [w139] -> w93 mode=indexing
      tunnel: w98 -> [w136]
      n25 = Unbundle By Name(w142) -> ("Format"=w140:T22, "Limit #"=w126:i32, "Ref Limit"=w127:bool, "Ref Type"=w128:enum32{"Current", "Specify"}, "Model"=w129:string, "Serial"=w130:string, "Run Type"=w131:enum32{"Most Recent", "Run #"}, "Run"=w132:i32, "Match Property"=w133:bool, "Property"=w134:string, "Property Value"=w135:string, "Upper"=w125:T23, "Lower"=w124:T23, "Nominal Values"=w123:dbl[])
      n26 = for {
        tunnel: w136 -> [w157]
        tunnel: w125 -> [w156] mode=indexing
        tunnel: [w152] -> w137 mode=indexing
        tunnel: w123 -> [w149]
        i -> [w148]
        n27 = Unbundle By Name(w156) -> ("Frequency"=w155:dbl, "Value"=w154:dbl, "Connected"=w153:bool)
        n28 = Index Array(array=w149, index=w148) -> (element=w146:dbl)
        n29 = Equal?(x=1.0, y=w146) -> (x = y?=w145:bool)
        n30 = Equal To 0?(x=w146) -> (x = 0?=w147:bool)
        n31 = Or(x=w145, y=w147) -> (x .or. y?=w143:bool)
        n32 = Select(t=nan, s=w143, f=w146) -> (s? t:f=w150:dbl)
        n33 = Bundle By Name(cluster=w157, "Frequency"=w155, "Value"=w154, "Connected"=w153, "Nominal Value"=w150) -> (w152:T19)
      }
      n34 = for {
        tunnel: w136 -> [w172]
        tunnel: w124 -> [w171] mode=indexing
        tunnel: [w167] -> w138 mode=indexing
        tunnel: w123 -> [w164]
        i -> [w163]
        n35 = Unbundle By Name(w171) -> ("Frequency"=w170:dbl, "Value"=w169:dbl, "Connected"=w168:bool)
        n36 = Index Array(array=w164, index=w163) -> (element=w158:dbl)
        n37 = Equal?(x=1.0, y=w158) -> (x = y?=w161:bool)
        n38 = Equal To 0?(x=w158) -> (x = 0?=w160:bool)
        n39 = Or(x=w161, y=w160) -> (x .or. y?=w159:bool)
        n40 = Select(t=nan, s=w159, f=w158) -> (s? t:f=w165:dbl)
        n41 = Bundle By Name(cluster=w172, "Frequency"=w170, "Value"=w169, "Connected"=w168, "Nominal Value"=w165) -> (w167:T19)
      }
      n42 = Bundle By Name(cluster=w141, "Format"=w140, "Limit #"=w126, "Ref Limit"=w127, "Ref Type"=w128, "Model"=w129, "Serial"=w130, "Run Type"=w131, "Run"=w132, "Match Property"=w133, "Property"=w134, "Property Value"=w135, "Upper"=w137, "Lower"=w138) -> (w139:T17)
    }
    n43 = case shown="\"S22\"" w95 {
      tunnel: [T20 {"Stimulus Port"=1, "Response Port"=1} ("Parameter") T20 {"Stimulus Port"=1, "Response Port"=2} ("Parameter") T20 {"Stimulus Port"=2, "Response Port"=1} ("Parameter") T20 {"Stimulus Port"=2, "Response Port"=2} ("Parameter")] -> w94
      frame "S11" {
      }
      frame "S21" {
      }
      frame "S12" {
      }
      frame "S22" {
      }
    }
    n44 = Bundle By Name(cluster=w97, "Parameter"=w94, "Limits"=w93) -> (w96:T15)
    n45 = Search 1D Array(1D array=w89, element=w88) -> (index of element=w87:i32)  [unwired: 1 out]
    n46 = case shown="Default" w87 {
      selector: w87 -> [w106 _]
      tunnel: w101 -> [w113 w122]
      tunnel: w96 -> [w110 w121]
      tunnel: w92 -> [w108 w119]
      tunnel: [w107 w117] -> w91
      tunnel: [w104 w116] -> w90
      tunnel: w89 -> [w104 w115]
      tunnel: w88 -> [w103 w114]
      frame Default {
        n47 = Index Array(array=w108, index=w106) -> (element=w112:T11)
        n48 = Unbundle By Name(w112) -> ("Parameters"=w111:T12)
        n49 = Build Array (concatenate)(w111, w110) -> (w109:T12)
        n50 = Bundle By Name(cluster=w113, "Channel"=w103, "Parameters"=w109) -> (w105:T11)
        n51 = Replace Array Subset(array=w108, new element=w105, index=w106) -> (w107:T5)
      }
      frame -1 {
        n52 = Build Array(w121) -> (w120:T12)
        n53 = Bundle By Name(cluster=w122, "Channel"=w114, "Parameters"=w120) -> (w118:T11)
        n54 = Build Array (concatenate)(w115, w114) -> (w116:i32[])
        n55 = Build Array (concatenate)(w119, w118) -> (w117:T5)
      }
    }
  }
  n56 = Or Array Elements(Boolean array=w2) -> (logical OR=w1:bool)
  n57 = Bundle By Name(cluster=w8, "Calibration.State"=w27, "Tag"=w31, "Stimulus"=w28, "Datasheets"=w29, "Display.Retain Settings"=w25, "Display.Lock Control"=w24, "Display.Plot Orientation"=w23, "Display.Formatted Data"=w1, "Calibration.State"=w18, "Auto Select"=FALSE, "Display.CH Controls"=w21, "Measurements"=w7) -> (→"S Parameter 3.2 - 4.1 Test Parameters":T1)
